vi "Read SequenceConfig.vi"(8 "error in (no error)":errorcluster, 11 "SequenceRepo in":refnum<class "SequenceRepo.lvclass">) -> (0 "error out":errorcluster, 2 "Sequence Config.lvclass":refnum<class "Sequence Config.lvclass">, 3 "SequenceRepo out":refnum<class "SequenceRepo.lvclass">)   [LabVIEW 2015, in "SequenceRepo.lvclass"]
uses:
  SequenceRepo.lvclass
  Prototype/classes/Sequence/Config/Sequence Config.lvclass
  SequenceRepo.lvclass/SequenceRepo.ctl
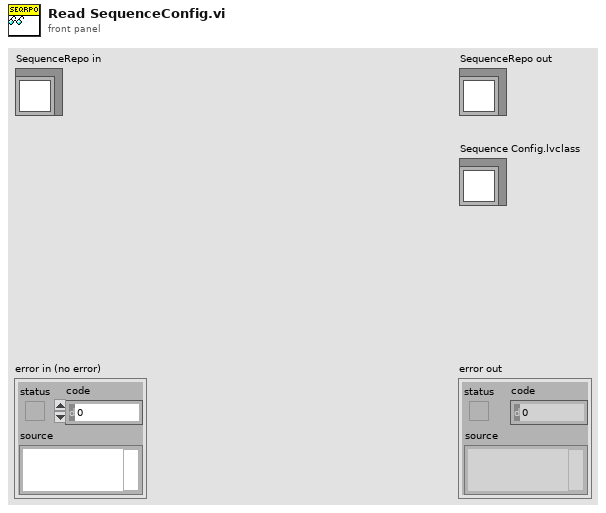
[diagram p1: front panel]
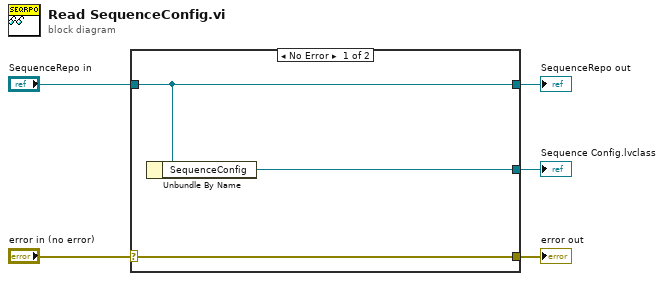
[diagram p0: block diagram]
diagram:
  n1 = case shown="No Error" "error in (no error)" {
    selector: "error in (no error)" -> [w8 w9]
    tunnel: [w8 w9] -> w4
    tunnel: [w7 w10] -> w2
    tunnel: "SequenceRepo in" -> [w7 w10]
    tunnel: [w6 _] -> w1
    frame No Error {
      n2 = Unbundle By Name(w7) -> ("SequenceConfig"=w6:refnum<class "Sequence Config.lvclass">)
    }
    frame Error {
    }
  }
  "error out" <- w4
  "SequenceRepo out" <- w2
  "Sequence Config.lvclass" <- w1
